vi "PH_gentec_Powermeter.get Energy.vi"(0 "i ref in":refnum<vi>, 2 "VISA resource in":refnum<visa-resource-name>, 5 "error in":errorcluster) -> (13 "Timeout":bool, 14 "i ref out":refnum<vi>, 17 "Error Message":string, 18 "Device Error out":errorcluster, 19 "error out":errorcluster)   [LabVIEW 2014, in "PH_gentec_Powermeter.lvlib"]
uses:
  PH_gentec_Powermeter.lvlib
  instr.lib/gentec-SOLO-PE/Driver/Type Defs/gentec-SOLO-PE.Enable Statistics.ctl
  PH_Basics/PH_Powermeter_BaseClass/PH_Powermeter_BaseClass.lvlib
  instr.lib/gentec-SOLO-PE/gentec-SOLO-PE - Driver.lvlib
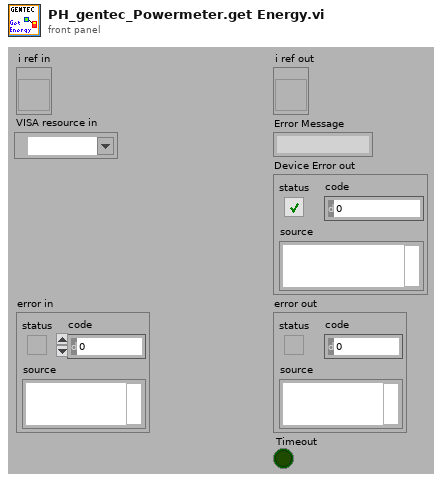
[diagram p1: front panel]
types:
  T1 = typedef "PH_Powermeter_BaseClass.lvlib/PH_Powermeter_BaseClass.i attribute.ctl" = cluster{"GUI References":T2, "Connection":T3, "Head Attributes":T5, "VISA resource":refnum<visa-resource-name>, "Energy":T6, "Service ID Energy":i32, "Wanted Settings":T7, "Current Settings":T7}
  T2 = typedef "PH_Powermeter_BaseClass.lvlib/PH_Powermeter_BaseClass.GUI Refs.ctl" = cluster{"Head Attributes":refnum<vi>, "Energy":refnum<vi>, "Connection":refnum<vi>, "VISA Resource":refnum<vi>, "Energy evolution":refnum<vi>, "Scaling Factor":refnum<vi>, "Range":refnum<vi>, "Wavelength":refnum<vi>, "Trigger Level":refnum<vi>, "Wanted Settings":refnum<vi>, "Current Settings":refnum<vi>}
  T3 = typedef "PH_Powermeter_BaseClass.lvlib/PH_Powermeter_BaseClass.Connection.ctl" = cluster{"failed checks":i8, "Timeout":bool, "Data read":string, "Failure":bool, "Error":bool, "State":T4}
  T4 = typedef "PH_Powermeter_BaseClass.lvlib/PH_Powermeter_BaseClass.State.ctl" = enum32{"off", "operating", "opened", "checked", "connected", "Sets to change", "running"}
  T5 = typedef "PH_Powermeter_BaseClass.lvlib/PH_Powermeter_BaseClass.Head Attributes.ctl" = cluster{"Instrument Type":string, "Head Version":string, "Head Name":string, "Serial Number":string, "Firmware":string, "Sensor Type":string, "MinimumRange":u32, "Maximum Range":u32, "Min Wavelength":i32, "Max Wavelength":i32}
  T6 = typedef "PH_Powermeter_BaseClass.lvlib/PH_Powermeter_BaseClass.Energy.ctl" = cluster{"current Value":dbl, "unscaled":dbl, "Scaling Factor":dbl}
  T7 = typedef "PH_Powermeter_BaseClass.lvlib/PH_gentec_BaseClass.Head Settings.ctl" = cluster{"Trigger Level":dbl, "Wavelength":u32, "Range":u32}
  T8 = typedef "PH_gentec_Powermeter.lvlib/PH_gentec_Powermeter.i attribute.ctl" = cluster{"GUI References":cluster{"delete":refnum<vi>, "start stop Statistics":refnum<vi>, "Statistic Data":refnum<vi>, "Configuration Values":refnum<vi>, "Set Zero":refnum<vi>, "Data Sampling Settings":refnum<vi>, "Wanted Sets":refnum<vi>, "Current Sets":refnum<vi>}, "Start Stop Statistics":bool, "Wanted Sets":T9, "Current Sets":T9}
  T9 = typedef "PH_gentec_Powermeter.lvlib/PH_gentec_Powermeter.Sets.ctl" = cluster{"Data Sampling Settings":T10, "Set Zero":bool}
  T10 = typedef "gentec-SOLO-PE - Driver.lvlib/gentec-SOLO-PE.Data Sampling Settings.ctl" = cluster{"Sample Rate":u32, "Sample Rate Unit":u32, "Sample Period":u32, "Sample Period Unit":u32, "Total Duration":u32, "Total Duration Unit":u32, "Time Stamp":u32}
  T11 = typedef "gentec-SOLO-PE - Driver.lvlib/gentec-SOLO-PE.Statistics Data.ctl" = cluster{"Current Value":dbl, "Maximum":dbl, "Minimum":dbl, "Average":dbl, "Standard Deviation":dbl, "RMS Stability":dbl, "PTP Stability":dbl, "Current Time In Period":u32, "Total Time in Period":u32, "Pulse Number":u32, "Total Pulses":u32, "Average Power":dbl, "Rep Rate":dbl, "Uncorrected Value":dbl}
  T12 = typedef "gentec-SOLO-PE - Driver.lvlib/gentec-SOLO-PE.Enable Statistics.ctl" = u32
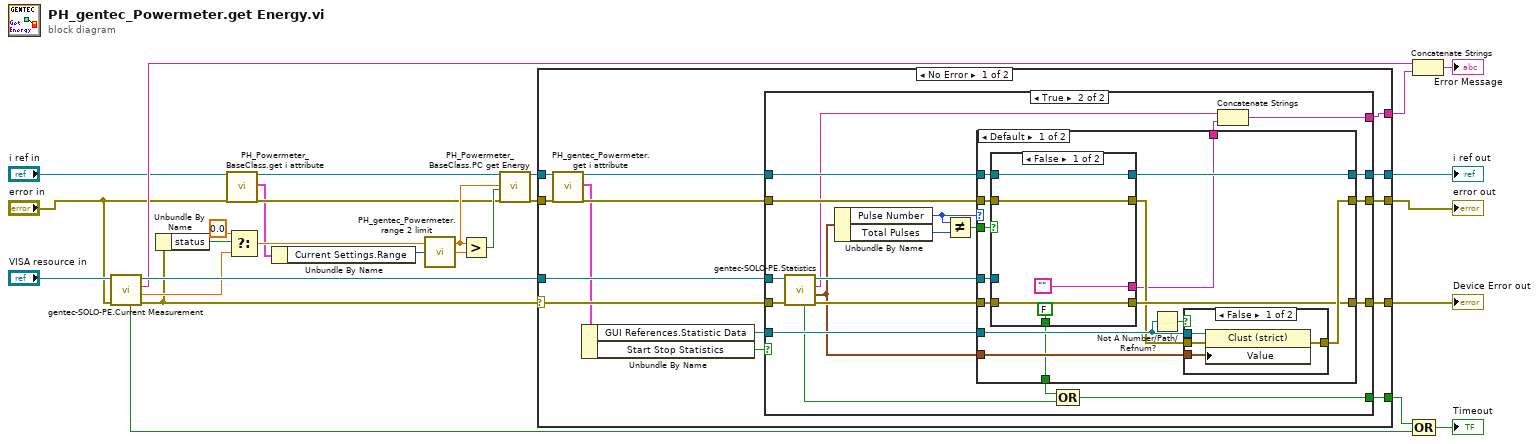
[diagram p0: block diagram]
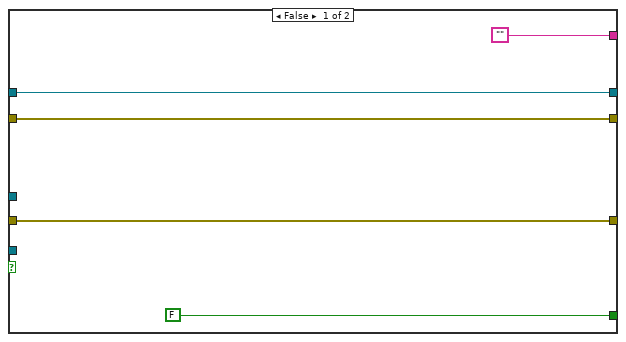
[diagram p2: hidden frame]
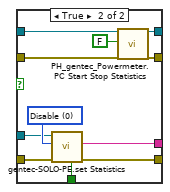
[diagram p3: hidden frame]
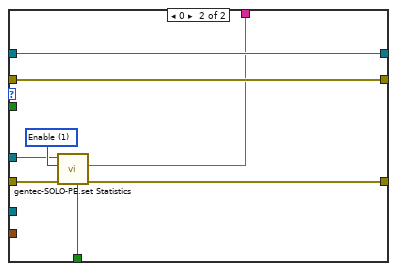
[diagram p5: hidden frame]
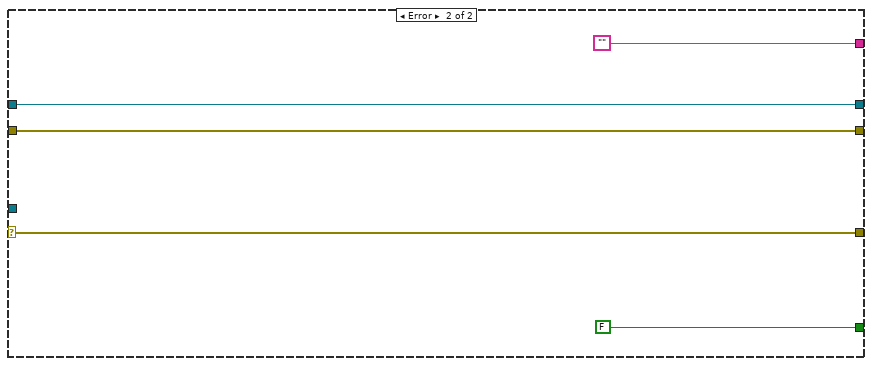
[diagram p6: hidden frame]
diagram:
  n1 = call "gentec-SOLO-PE.Current Measurement.vi"("error in (no error)"="error in", "VISA Refnum in"="VISA resource in") -> ("error out"=w15:errorcluster, "Uncorrected Value [J]"=w17:dbl, "Error"=w9:string, "VISA Refnum out"=w26:refnum<visa-resource-name>, "Timeout"=w11:bool)  [unwired: 4 in, 1 out]
  n2 = Unbundle By Name(w15) -> ("status"=w19:bool)
  n3 = call "PH_Powermeter_BaseClass.get i attribute.vi"("i ref in"="i ref in", "error in (no error)"="error in") -> ("i ref out"=w5:refnum<vi>, "i attribute"=w4:T1, "error out"=w6:errorcluster)  [unwired: 15 in]
  n4 = Select(t=0.0, s=w19, f=w17) -> (s? t:f=w16:dbl)
  n5 = Unbundle By Name(w4) -> ("Current Settings.Range"=w3:u32)
  n6 = call "PH_gentec_Powermeter.range 2 limit.vi"("Range"=w3) -> ("limit"=w21:dbl)
  n7 = Greater?(x=w16, y=w21) -> (0:w20:bool)
  n8 = call "PH_Powermeter_BaseClass.PC get Energy.vi"("i ref in"=w5, "unscaled Energy [J]"=w16, "Out of range?"=w20, "error in"=w6) -> ("i ref out"=w22:refnum<vi>, "error out"=w23:errorcluster)  [unwired: 14 in]
  n9 = case shown="No Error" w15 {
    selector: w15 -> [w36 w111]
    tunnel: w26 -> [w40 _]
    tunnel: [w39 w111] -> w25
    tunnel: [w38 w112] -> w13
    tunnel: [w37 w113] -> w14
    tunnel: w23 -> [w30 w112]
    tunnel: w22 -> [w29 w113]
    tunnel: [w35 FALSE] -> w10
    tunnel: [w34 ""] -> w7
    frame No Error {
      n10 = call "PH_gentec_Powermeter.get i attribute.vi"("i ref in"=w29, "error in (no error)"=w30) -> ("i ref out"=w28:refnum<vi>, "i attribute"=w27:T8, "error out"=w31:errorcluster)  [unwired: 15 in]
      n11 = Unbundle By Name(w27) -> ("GUI References.Statistic Data"=w33:refnum<vi>, "Start Stop Statistics"=w32:bool)
      n12 = case shown="True" w32 {
        tunnel: w36 -> [w45 w65]
        tunnel: [w45 w61] -> w39
        tunnel: w40 -> [_ w64]
        tunnel: w33 -> [_ w58]
        tunnel: w31 -> [w43 w57]
        tunnel: [w43 w56] -> w38
        tunnel: w28 -> [w44 w54]
        tunnel: [w44 w53] -> w37
        tunnel: [FALSE w49] -> w35
        tunnel: ["" w46] -> w34
        frame False {
        }
        frame True {
          n13 = call "gentec-SOLO-PE.Statistics.vi"("error in (no error)"=w65, "VISA Refnum in"=w64) -> ("error out"=w62:errorcluster, "Statistic Data"=w52:T11, "Error"=w48:string, "VISA Refnum out"=w60:refnum<visa-resource-name>, "Timeout"=w51:bool)  [unwired: 5 in]
          n14 = Unbundle By Name(w52) -> ("Pulse Number"=w59:u32, "Total Pulses"=w63:u32)
          n15 = Not Equal?(x=w59, y=w63) -> (x != y?=w55:bool)
          n16 = case shown="Default" w59 {
            tunnel: w62 -> [w74 w108]
            tunnel: [w73 w107] -> w61
            tunnel: w60 -> [w75 w105]
            tunnel: w52 -> [w78 _]
            tunnel: w58 -> [w77 _]
            tunnel: w57 -> [w70 w103]
            tunnel: [w76 w103] -> w56
            tunnel: w55 -> [w72 _]
            tunnel: w54 -> [w71 w104]
            tunnel: [w69 w104] -> w53
            tunnel: [w67 w102] -> w50
            tunnel: [w66 w101] -> w47
            frame Default {
              n17 = case shown="False" w72 {
                tunnel: w75 -> [_ w94]
                tunnel: w74 -> [w84 w93]
                tunnel: [w84 w92] -> w73
                tunnel: w71 -> [w83 w90]
                tunnel: w70 -> [w82 w89]
                tunnel: [w83 w88] -> w69
                tunnel: [w82 w87] -> w68
                tunnel: [FALSE ("Timeout") w86] -> w67
                tunnel: ["" w85] -> w66
                frame False {
                }
                frame True {
                  w95 = T12 0 items=["Disable", "Enable", "Reset", "Read"] ("Operation")
                  n18 = call "gentec-SOLO-PE.set Statistics.vi"("error in (no error)"=w93, "Enable Statistics"=w95, "VISA Refnum in"=w94) -> ("error out"=w92:errorcluster, "Error"=w85:string, "Timeout"=w86:bool)  [unwired: 4 in, 2 out]
                  n19 = call "PH_gentec_Powermeter.PC Start Stop Statistics.vi"("VI in"=w90, "Start / Stop Statistics"=FALSE ("Start / Stop"), "error in (no error)"=w89) -> ("VI out"=w88:refnum<vi>, "error out"=w87:errorcluster)  [unwired: 15 in]
                }
              }
              n20 = Not A Number/Path/Refnum?(number/path/refnum=w77) -> (NaN/Path/Refnum?=w79:bool)
              n21 = case shown="False" w79 {
                tunnel: [w99 w100] -> w76
                tunnel: w78 -> [w98 _]
                tunnel: w68 -> [w97 w100]
                tunnel: w77 -> [w96 _]
                frame False {
                  n22 = property class="Clust (strict)"(reference=w96, error in=w97, "Value"=w98) -> (error out=w99:errorcluster)  [unwired: 1 out]
                }
                frame True {
                }
              }
            }
            frame 0 {
              w106 = T12 1 items=["Disable", "Enable", "Reset", "Read"] ("Operation")
              n23 = call "gentec-SOLO-PE.set Statistics.vi"("error in (no error)"=w108, "Enable Statistics"=w106, "VISA Refnum in"=w105) -> ("error out"=w107:errorcluster, "Error"=w101:string, "Timeout"=w102:bool)  [unwired: 4 in, 2 out]
            }
          }
          n24 = Compound Arithmetic op=OR(w50, w51) -> (w49:bool)
          n25 = Concatenate Strings(w48, w47) -> (w46:string)
        }
      }
    }
    frame Error {
    }
  }
  "i ref out" <- w14
  "error out" <- w13
  "Device Error out" <- w25
  n26 = Concatenate Strings(w9, w7) -> (→"Error Message":string)
  n27 = Compound Arithmetic op=OR(w10, w11) -> (→"Timeout":bool)
